vi "1D数组排序[CSG 实部,虚部].vi"(8 "error in (no error)":errorcluster caption="错误输入（无错误）", 9 "升降序":enum16{"升序", "降序"}(ring), 11 "输入数组":csg[](array[numeric])) -> (0 "error out":errorcluster caption="错误输出", 2 "排序后索引":i32[](array[numeric]), 3 "排序后数组":csg[](array[numeric]) format="%.2f")   [LabVIEW 2020]
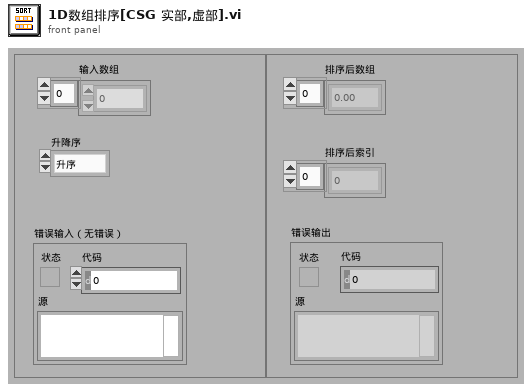
[diagram p1: front panel]
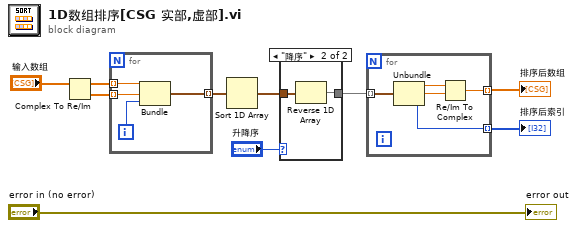
[diagram p0: block diagram]
diagram:
  n1 = Complex To Re/Im(x + iy="输入数组") -> (x=w8:sgl[], y=w7:sgl[])
  n2 = for {
    tunnel: w8 -> [w14] mode=indexing
    tunnel: w7 -> [w12] mode=indexing
    tunnel: [w13] -> w9 mode=indexing
    i -> [w11]
    n3 = Bundle("数值"=w14, "数值"=w12, w11) -> (w13:cluster{"数值":sgl, "数值":sgl, i32})  [unwired: 1 in]
  }
  n4 = Sort 1D Array(array=w9) -> (sorted array=w2:cluster{"数值":sgl, "数值":sgl, i32}[])
  n5 = case shown="\"降序\"" "升降序" {
    tunnel: w2 -> [w15 w17]
    tunnel: [w15 w16] -> w1
    frame "升序", Default {
    }
    frame "降序" {
      n6 = Reverse 1D Array(array=w17) -> (reversed array=w16:cluster{"数值":sgl, "数值":sgl, i32}[])
    }
  }
  n7 = for {
    tunnel: w1 -> [w22] mode=indexing
    tunnel: [w19] -> w5 mode=indexing
    tunnel: [w18] -> w4 mode=indexing
    n8 = Unbundle(w22) -> ("数值"=w21:sgl, "数值"=w20:sgl, w18:i32)
    n9 = Re/Im To Complex(1:w20, 2:w21) -> (0:w19:csg)
  }
  "排序后数组" <- w5
  "排序后索引" <- w4
  "error out" <- "error in (no error)"
